vi "ReceiveStringCheck.vi"(1 "VCI_CAN_OBJ_R":T1) -> (0 "约定ID":string)   [LabVIEW 2013]
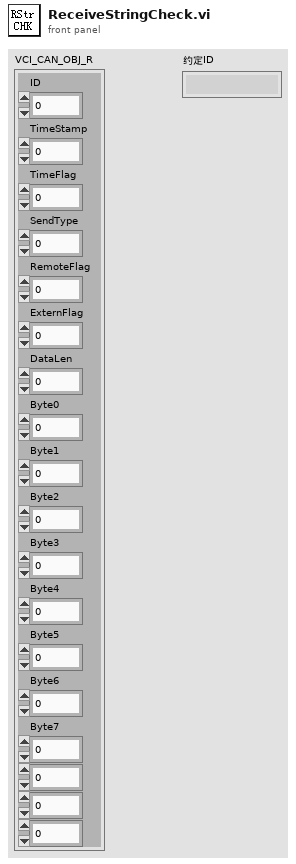
[diagram p1: front panel]
types:
  T1 = cluster{"ID":u32, "TimeStamp":u32, "TimeFlag":u8, "SendType":u8, "RemoteFlag":u8, "ExternFlag":u8, "DataLen":u8, "Byte0":u8, "Byte1":u8, "Byte2":u8, "Byte3":u8, "Byte4":u8, "Byte5":u8, "Byte6":u8, "Byte7":u8, u8, u8, u8}
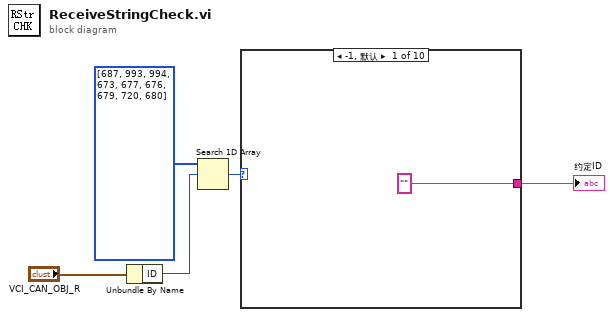
[diagram p0: block diagram]
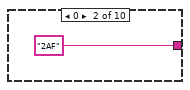
[diagram p2: hidden frame]
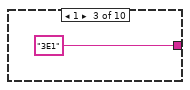
[diagram p3: hidden frame]
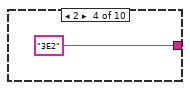
[diagram p4: hidden frame]
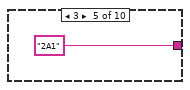
[diagram p5: hidden frame]
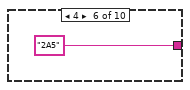
[diagram p6: hidden frame]
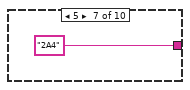
[diagram p7: hidden frame]
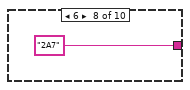
[diagram p8: hidden frame]
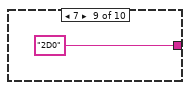
[diagram p9: hidden frame]
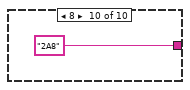
[diagram p10: hidden frame]
diagram:
  n1 = Unbundle By Name("VCI_CAN_OBJ_R") -> ("ID"=w4:u32)
  n2 = Search 1D Array(1D array=i32[] [687, 993, 994, 673, 677, 676, 679, 720, 680], element=w4) -> (index of element=w3:i32)  [unwired: 1 in]
  n3 = case shown="-1, 默认" w3 {
    tunnel: ["" "2AF" "3E1" "3E2" "2A1" "2A5" "2A4" "2A7" "2D0" "2A8"] -> w2
    frame -1, Default {
    }
    frame 0 {
    }
    frame 1 {
    }
    frame 2 {
    }
    frame 3 {
    }
    frame 4 {
    }
    frame 5 {
    }
    frame 6 {
    }
    frame 7 {
    }
    frame 8 {
    }
  }
  "约定ID" <- w2
